vi "Hinge_Loss.vi"(8 "error in (no error)":errorcluster caption="entrée d'erreur (pas d'erreur)", 9 "pred_decision":string[][](array[string]), 10 "y_true":string[][](array[string]), 11 "hinge_loss":cluster{"labels":i32[], "sample_weight":dbl[]}) -> (0 "error out":errorcluster caption="sortie d'erreur", 3 "Score":string)   [LabVIEW 2020]
doc: "Average hinge loss (non-regularized)\n\nIn binary class case, assuming labels in y_true are encoded with +1 and -1, when a prediction mistake is made, margin = y_true * pred_decision is always negative (since the signs disagree), implying 1 - margin is always greater than 1. The cumulated hinge loss is therefore an upper bound of the number of mistakes made by the classifier.\n\nIn multiclass case, the function expects that either all the labels are included in y_true or an optional labels argument is provided which contains all the labels. The multilabel margin is calculated according to Crammer-Singer’s method. As in the binary case, the cumulated hinge loss is an upper bound of the number of mistakes made by the classifier.\n\n\n\nParameters : \n\n- y_true : array, shape = [n_samples]\nTrue target, consisting of integers of two values. The positive label must be greater than the negative label.\n\n- pred_decision : array, shape = [n_samples] or [n_samples, n_classes]\nPredicted decisions, as output by decision_function (floats).\n\n- labels : array, optional, default None\nContains all the labels for the problem. Used in multiclass hinge loss.\n\n- sample_weight : array-like of shape (n_samples,), default=None\nSample weights.\n\nReturns : \n\n- loss : float"
uses:
  Hinge_Loss.lvclass
panel:
  out "Hinge_Loss.lvclass":refnum<class "Hinge_Loss.lvclass">
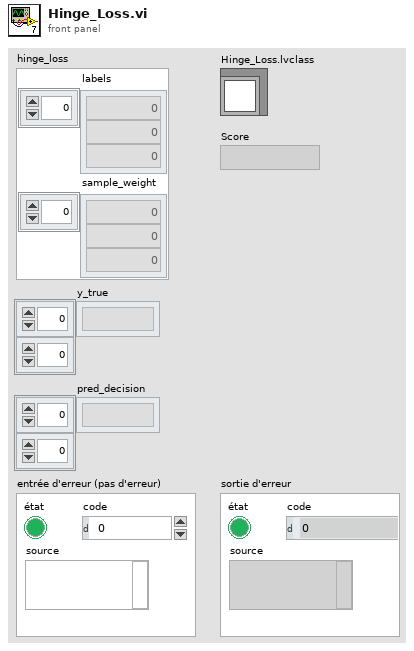
[diagram p1: front panel]
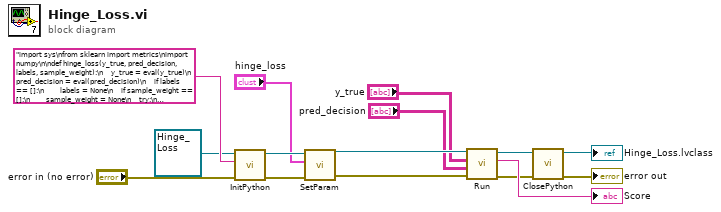
[diagram p0: block diagram]
diagram:
  n1 = call-dynamic "InitPython.vi"("error in (no error)"="error in (no error)", "Python Instruction"="import sys\nfrom sklearn import metrics\nimport numpy\n\ndef hinge_loss(y_true, pred_decision, labels, sample_weight):\n    y_true = eval(y_true)\n    pred_decision = eval(pred_decision)\n    if labels == []:\n        labels = None\n    if sample_weight == []:\n        sample_weight = None\n    try:\n        hinge_loss = metrics.hinge_loss(y_true, pred_decision, labels, sample_weight)\n        hinge_loss = hinge_loss.tolist()\n        return str(hinge_loss)\n    except:\n        erreur = sys.exc_info()\n        typerr = u\"%s\" % (erreur[0])\n        typerr = typerr[typerr.find(\"'\")+1:typerr.rfind(\"'\")]\n        msgerr = u\"%s\" % (erreur[1])\n        message = str('/!\\\\ {0} : {1}'. format(typerr,msgerr))\n        return message", "Scikit-learn en entrée"=refnum<class "Hinge_Loss.lvclass"> refnum ("Hinge_Loss.lvclass")) -> ("error out"=w9:errorcluster, "Scikit-learn en sortie"=w11:refnum<class "Hinge_Loss.lvclass">)  [unwired: 7 in]
  n2 = call-dynamic "SetParam.vi"("error in (no error)"=w9, "hinge_loss"="hinge_loss", "Hinge_Loss.lvclass"=w11) -> ("error out"=w7:errorcluster, "Hinge_Loss.lvclass"=w8:refnum<class "Hinge_Loss.lvclass">)  [unwired: 7 in]
  n3 = call-dynamic "Run.vi"("error in (no error)"=w7, "pred_decision"="pred_decision", "y_true"="y_true", "Hinge_Loss.lvclass"=w8) -> ("error out"=w4:errorcluster, "String Data"=→"Score":string, "Hinge_Loss.lvclass"=w6:refnum<class "Hinge_Loss.lvclass">)  [unwired: 5 in]
  n4 = call-dynamic "ClosePython.vi"("error in (no error)"=w4, "Scikit-learn en entrée"=w6) -> ("error out"=→"error out":errorcluster, "Scikit-learn en sortie"=→"Hinge_Loss.lvclass":refnum<class "Hinge_Loss.lvclass">)  [unwired: 8 in]
